vi "1D Histogram or PDF, unweighted_PN.vi"(0 "Nbins":i32, 3 "Mean shift":bool, 4 "mean":dbl, 7 "max":dbl, 8 "Current block no.":i32, 9 "min":dbl, 11 "Shift SumW in":dbl, 12 "PDF":bool=TRUE, 13 "Shift PDF in":dbl[](array[numeric]), 16 "1D data":dbl[](array[numeric])) -> (20 "1D histogram or PDF":dbl[](array[numeric]), 22 "bin centre vals.":dbl[](array[numeric]), 24 "bin width":dbl, 26 "Shift SumW out":dbl, 27 "Shift PDF out":dbl[](array[numeric]))   [LabVIEW 2020]
panel:
  out "1D histogram or PDF":cluster{"UbinC":dbl[], dbl[]}(graph)
  # "N.B. The values of Umax, Umin, Umean MUST be those of the ENTIRE dataset (i.e. all blocks) otherwise this routine will be inconsistent."
  # "Paul Nathan 03/10/2012"
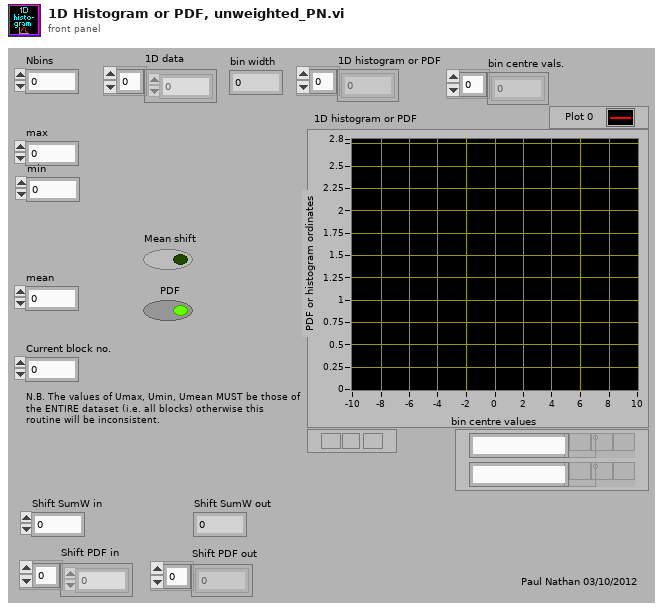
[diagram p1: front panel]
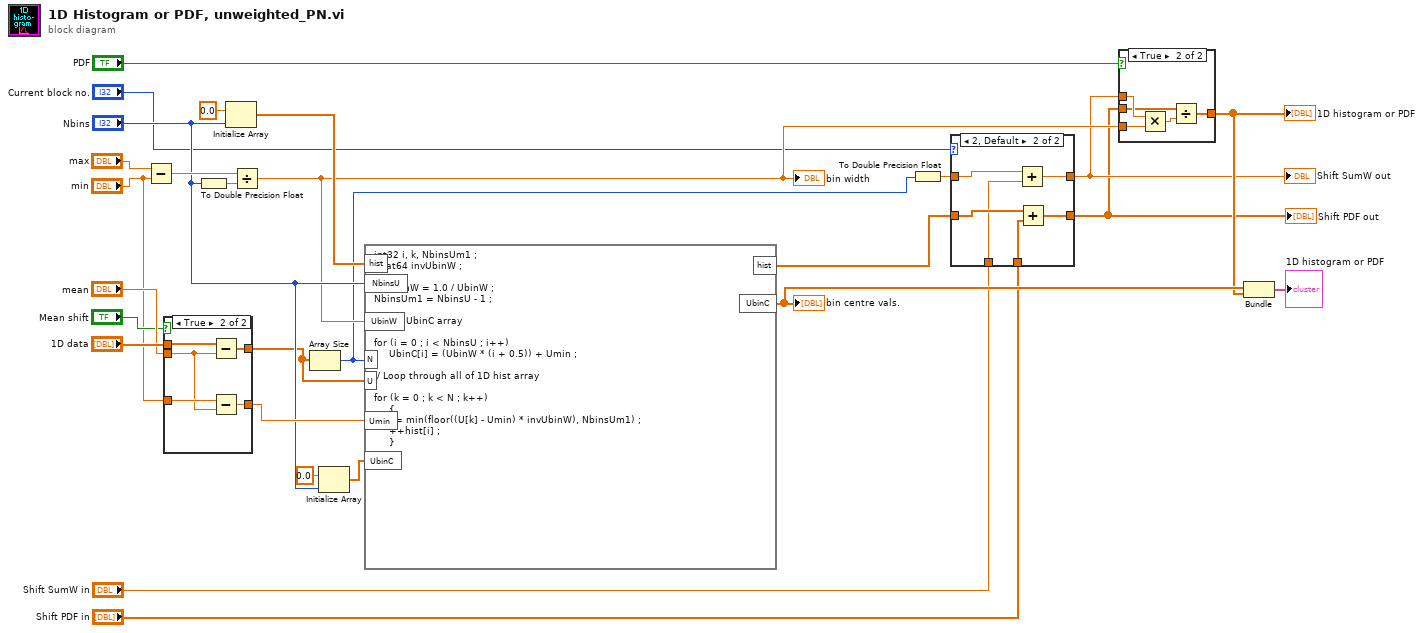
[diagram p0: block diagram]
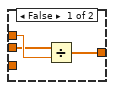
[diagram p3: hidden frame]
diagram:
  n1 = Subtract(x="max", y="min") -> (x-y=w19:dbl)
  n2 = case shown="True" "Mean shift" {
    tunnel: "1D data" -> [w29 w34]
    tunnel: "mean" -> [_ w31]
    tunnel: [w29 w33] -> w15
    tunnel: "min" -> [w28 w32]
    tunnel: [w28 w30] -> w18
    frame False {
    }
    frame True {
      n3 = Subtract(x=w34, y=w31) -> (x-y=w33:dbl[])
      n4 = Subtract(x=w32, y=w31) -> (x-y=w30:dbl)
    }
  }
  n5 = To Double Precision Float(number="Nbins") -> (double precision float=w27:dbl)
  n6 = Initialize Array(0.0 ("element"), "Nbins") -> (w22:dbl[])
  n7 = Divide(x=w19, y=w27) -> (x/y=w12:dbl)
  "bin width" <- w12
  n8 = Array Size(array=w15) -> (size(s)=w2:i32)
  n9 = Initialize Array(0.0 ("element"), "Nbins") -> (w14:dbl[])
  n10 = formula code="int32 i, k, NbinsUm1 ;\nfloat64 invUbinW ;\n\ninvUbinW = 1.0 / UbinW ;\nNbinsUm1 = NbinsU - 1 ;\n\n// Calc UbinC array\n\nfor (i = 0 ; i < NbinsU ; i++)\n     UbinC[i] = (UbinW * (i + 0.5)) + Umin ;\n\n// Loop through all of 1D hist array \n\nfor (k = 0 ; k < N ; k++)\n     {\n     i = min(floor((U[k] - Umin) * invUbinW), NbinsUm1) ;\n     ++hist[i] ;\n     }"("NbinsU"="Nbins", "N"=w2, "UbinW"=w12, "hist"=w22, "Umin"=w18, "UbinC"=w14, "U"=w15) -> ("hist"=w7:dbl[], "UbinC"=w11:dbl[])
  "bin centre vals." <- w11
  n11 = To Double Precision Float(number=w2) -> (double precision float=w1:dbl)
  n12 = case shown="2, Default" "Current block no." {
    tunnel: [w36 w41] -> w5
    tunnel: w7 -> [w36 w40]
    tunnel: w1 -> [w35 w39]
    tunnel: [w35 w42] -> w6
    tunnel: "Shift PDF in" -> [_ w38]
    tunnel: "Shift SumW in" -> [_ w37]
    frame 1 {
    }
    frame 2, Default {
      n13 = Add(x=w39, y=w37) -> (x+y=w42:dbl)
      n14 = Add(x=w40, y=w38) -> (x+y=w41:dbl[])
    }
  }
  "Shift PDF out" <- w5
  "Shift SumW out" <- w6
  n15 = case shown="True" "PDF" {
    tunnel: w12 -> [_ w49]
    tunnel: w6 -> [w45 w50]
    tunnel: w5 -> [w44 w48]
    tunnel: [w43 w46] -> w10
    frame False {
      n16 = Divide(x=w44, y=w45) -> (x/y=w43:dbl[])
    }
    frame True {
      n17 = Multiply(x=w50, y=w49) -> (x*y=w47:dbl)
      n18 = Divide(x=w48, y=w47) -> (x/y=w46:dbl[])
    }
  }
  "1D histogram or PDF" <- w10
  n19 = Bundle("UbinC"=w11, w10) -> (→"1D histogram or PDF":cluster{"UbinC":dbl[], dbl[]})  [unwired: 1 out]
